vi "merFISH_check_stability.vi"(5 "queue ASI stage":refnum<queue>, 6 "error in":errorcluster, 7 "Measure QPD":bool caption="Calibration", 8 "Data cluster":T1, 9 "queue piezo":refnum<queue>) -> (0 "error out":errorcluster)   [LabVIEW 2015]
uses:
  CONTROLS/Q_MCL_piezo_element.ctl
  CONTROLS/Q_ASI_stage_element.ctl
  GLOBAL/Global_MCL_piezo.vi
  GLOBAL/Global_ABORT.vi
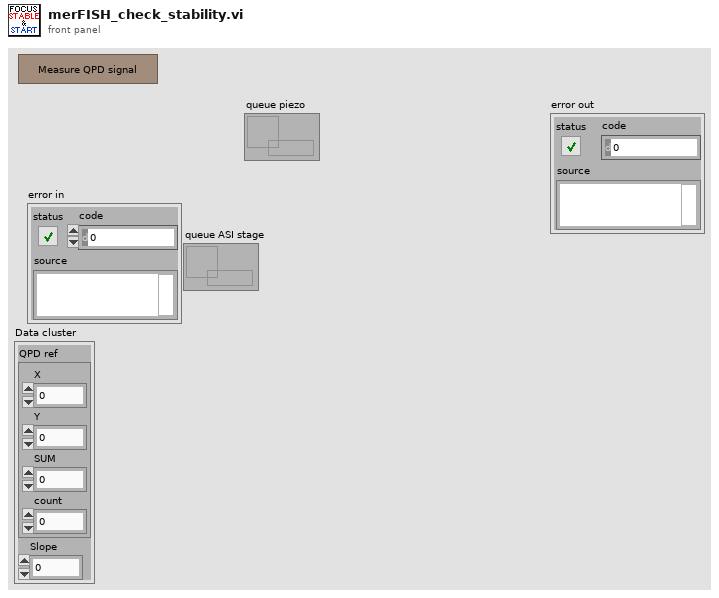
[diagram p1: front panel]
types:
  T1 = cluster{"QPD ref":cluster{"X":sgl, "Y":sgl, "SUM":sgl, "count":u32}, "Slope":dbl}
  T2 = cluster{"X":sgl, "Y":sgl, "SUM":sgl, "count":u32}
  T3 = typedef "Q_MCL_piezo_element.ctl" = cluster{"variant":variant, "Instruction":enum16{"Piezo_idle", "Piezo_initialize", "Piezo_error", "Piezo_security_stop", "Piezo_read_z", "Piezo_move_z", "Piezo_keyboard_move", "Piezo_close_autofocus_calibration_ramp", "Piezo_change_init_state", "Piezo_init_autofocus", "Piezo_init_autofocus_merFISH_TL", "Piezo_autofocus", "Piezo_autofocus_merFISH_TL", "Piezo_stop_autofocus", "Piezo_stop_autofocus_merFISH_TL", "Piezo_autofocus_lost", "Piezo_resume_autofocus_merFISH_TL", "Piezo_check_z_position_merFISH_TL", "Piezo_init_ramp", "Piezo_move_z_ramp", "Piezo_close_ramp", "Piezo_close_merFISH", "Piezo_stop"}}
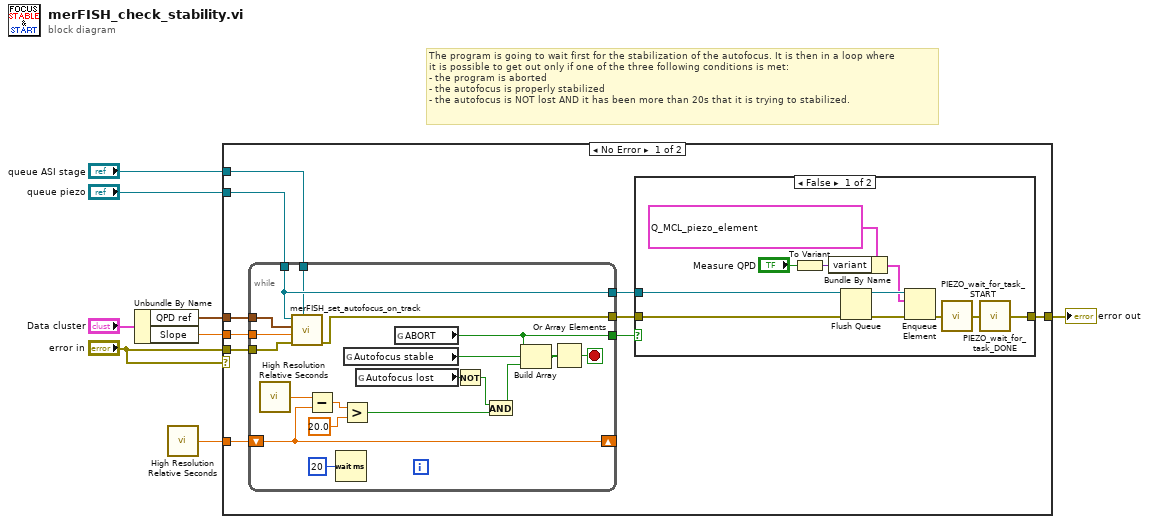
[diagram p0: block diagram]
diagram:
  # "The program is going to wait first for the stabilization of the autofocus. It is then in a loop where \nit is possible to get out only if one of the three following conditions is met:\n- the program is aborted\n- the autofocus is properly stabilized\n- the autofocus is NOT lost AND it has been more than 20s that it is trying to stabilized."
  n1 = Unbundle By Name("Data cluster") -> ("QPD ref"=w2:T2, "Slope"=w3:dbl)
  n2 = call <vilib>:"High Resolution Relative Seconds.vi"() -> ("relative seconds"=w4:dbl)
  n3 = case shown="No Error" "error in" {
    tunnel: "error in" -> [w18 w50]
    tunnel: [w17 w50] -> w8
    tunnel: "queue piezo" -> [w15 _]
    tunnel: w2 -> [w13 _]
    tunnel: w3 -> [w12 _]
    tunnel: "queue ASI stage" -> [w11 _]
    tunnel: w4 -> [w10 _]
    frame No Error {
      n4 = while {
        tunnel: w18 -> [w48]
        tunnel: [w44] -> w9
        tunnel: [w34] -> w16
        tunnel: w15 -> [w47]
        tunnel: [w47] -> w14
        tunnel: w13 -> [w45]
        tunnel: w12 -> [w46]
        tunnel: w11 -> [w43]
        shift-right: [w31] -> _
        shift-left: w10 -> [w31]
        stop <- w32 stop-if-true
        n5 = call <vilib>:"High Resolution Relative Seconds.vi"() -> ("relative seconds"=w42:dbl)
        n6 = call "merFISH_set_autofocus_on_track.vi"("queue ASI stage"=w43, "error in"=w48, "Slope"=w46, "QPD ref"=w45, "queue piezo"=w47) -> ("error out"=w44:errorcluster)  [unwired: 4 in]
        n7 = Subtract(x=w42, y=w31) -> (x-y=w41:dbl)
        n8 = Wait (ms)(milliseconds to wait=u32 20) -> ()  [unwired: 1 out]
        n9 = Greater?(x=w41, y=20.0) -> (0:w37:bool)
        n10 = global read "Global_MCL_piezo.vi" "Autofocus stable"() -> (w35:bool)
        n11 = global read "Global_MCL_piezo.vi" "Autofocus lost"() -> (w38:bool)
        n12 = global read "Global_ABORT.vi" "ABORT"() -> (w34:bool)
        n13 = Not(x=w38) -> (.not. x?=w39:bool)
        n14 = And(x=w39, y=w37) -> (x .and. y?=w36:bool)
        n15 = Build Array(w34, w35, w36) -> (w33:bool[])
        n16 = Or Array Elements(Boolean array=w33) -> (logical OR=w32:bool)
      }
      n17 = case shown="False" w16 {
        tunnel: w9 -> [w20 w30]
        tunnel: [w19 w30] -> w17
        tunnel: w14 -> [w21 _]
        frame False {
          n18 = To Variant(anything="Measure QPD") -> (Variant=w24:variant)
          n19 = Bundle By Name(cluster=T3 {"variant"=variant, "Instruction"=enum."Piezo_stop_autofocus_merFISH_TL"} ("element"), "variant"=w24) -> (w22:T3)
          n20 = Flush Queue(queue=w21, error in (no error)=w20) -> (queue out=w26:refnum<queue>, error out=w27:errorcluster)  [unwired: 1 out]
          n21 = Enqueue Element(queue=w26, element=w22, error in (no error)=w27) -> (error out=w28:errorcluster)  [unwired: 1 in, 2 out]
          n22 = call "PIEZO_wait_for_task_START.vi"("error in"=w28) -> ("error out"=w29:errorcluster)
          n23 = call "PIEZO_wait_for_task_DONE.vi"("error in"=w29) -> ("error out"=w19:errorcluster)
        }
        frame True {
        }
      }
    }
    frame Error {
    }
  }
  "error out" <- w8
